vi "ListDiagrams.vi"(6 "diagram indices":i32[](array[numeric]), 8 "error in":errorcluster, 11 "CaseStructure in":refnum<class "CaseStructure.lvclass">) -> (0 "error out":errorcluster, 3 "CaseStructure out":refnum<class "CaseStructure.lvclass">, 5 "default":string, 7 "diagrams":string)   [LabVIEW 2014, in "Raspberry Pi Compatible Compiler for LabVIEW.lvlib" / "CaseStructure.lvclass"]
uses:
  CaseStructure.lvclass
  Python/Parsing/ListTypesTD.ctl
  Python/Parsing/Python Functions.lvlib
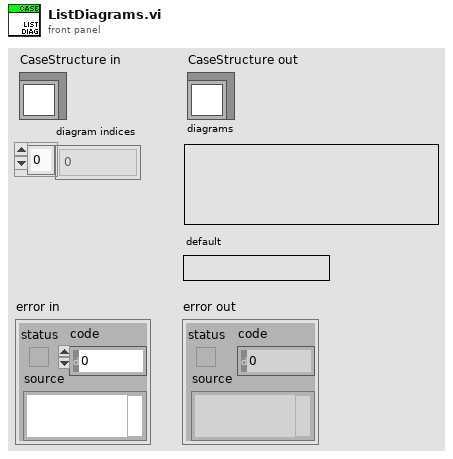
[diagram p1: front panel]
types:
  T1 = typedef "Raspberry Pi Compatible Compiler for LabVIEW.lvlib/Python Functions.lvlib/ListTypesTD.ctl" = enum16{"list", "tuple", "parameter list", "output list", "return values"}
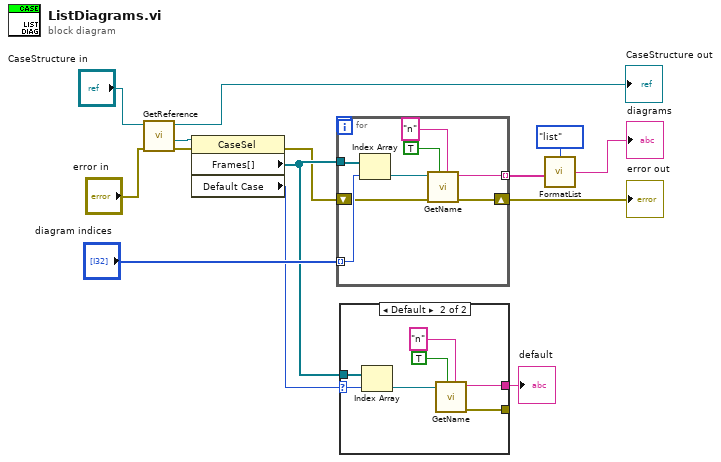
[diagram p0: block diagram]
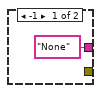
[diagram p2: hidden frame]
diagram:
  n1 = call "GetReference.vi"("error in"="error in", "CaseStructure in"="CaseStructure in") -> ("error out"=w10:errorcluster, "reference out"=w11:refnum<vi>, "CaseStructure out"=→"CaseStructure out":refnum<class "CaseStructure.lvclass">)  [unwired: 7 in]
  n2 = property class="CaseSel"(reference=w11, error in=w10) -> (error out=w3:errorcluster, "Frames[]"=w5:refnum<vi>[], "Default Case"=w4:i32)  [unwired: 1 out]
  n3 = for {
    tunnel: w5 -> [w22]
    tunnel: "diagram indices" -> [w21] mode=indexing
    shift-right: [w18] -> w2
    shift-left: w3 -> [w19]
    tunnel: [w15] -> w8 mode=indexing
    n4 = Index Array(array=w22, index=w21) -> (element=w20:refnum<vi>)
    n5 = call "GetName.vi"("base name"="n", "add self"=TRUE, "error in"=w19, "GObj Refnum"=w20) -> ("error out"=w18:errorcluster, "name"=w15:string)  [unwired: 5 in, 1 out]
  }
  "error out" <- w2
  n6 = case shown="Default" w4 {
    selector: w4 -> [_ w30]
    tunnel: w5 -> [_ w29]
    tunnel: [_ w25] -> _
    tunnel: ["None" ("name") w24] -> w1
    frame -1 {
    }
    frame Default {
      n7 = Index Array(array=w29, index=w30) -> (element=w26:refnum<vi>)
      n8 = call "GetName.vi"("base name"="n", "add self"=TRUE, "GObj Refnum"=w26) -> ("error out"=w25:errorcluster, "name"=w24:string)  [unwired: 6 in, 1 out]
    }
  }
  "default" <- w1
  n9 = call "FormatList.vi"("values"=w8, "type"=ListTypesTD."list") -> ("python object"=→"diagrams":string)
